vi "SQLite Gen Std.Insert Statement.vi"(10 "Field Name":string[](array[string]), 11 "Table Name":string) -> (3 "Insert Statement":string)   [LabVIEW 2021, in "EDT SQLite+.lvlib"]
uses:
  EDT SQLite+.lvlib
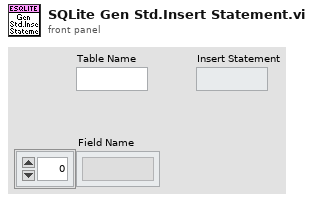
[diagram p1: front panel]
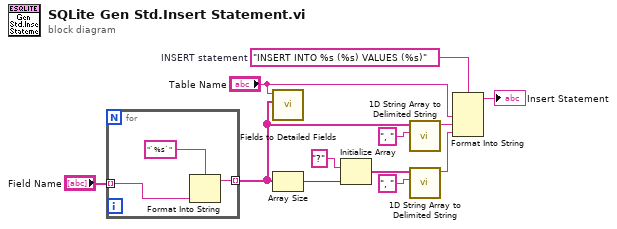
[diagram p0: block diagram]
diagram:
  w4 = "INSERT INTO %s (%s) VALUES (%s)"  # INSERT statement
  n1 = for {
    tunnel: "Field Name" -> [w14] mode=indexing
    tunnel: [w13] -> w1 mode=indexing
    n2 = Format Into String(format string="`%s`", w14) -> (resulting string=w13:string)  [unwired: 2 in, 1 out]
  }
  n3 = call "Fields to Detailed Fields.vi"("Fields"=w1, "Table Name"="Table Name") -> ()  [unwired: 9 in, 1 out]
  n4 = Array Size(array=w1) -> (size(s)=w8:i32)
  n5 = Initialize Array("?", w8) -> (w11:string[])
  n6 = call <vilib>:"1D String Array to Delimited String.vi"("delimiter"=", ", "string array"=w1) -> ("delimited string"=w6:string)  [unwired: 9 in]
  n7 = call <vilib>:"1D String Array to Delimited String.vi"("delimiter"=", ", "string array"=w11) -> ("delimited string"=w12:string)  [unwired: 9 in]
  n8 = Format Into String(format string=w4, "Table Name", w6, w12) -> (resulting string=→"Insert Statement":string)  [unwired: 2 in, 1 out]
